vi "Testing.vi"() -> ()   [LabVIEW 2016, in "User Interface.lvlib"]
uses:
  User Interface.lvlib
  <vilib>/Utility/miscctls.llb/LVPointTypeDef.ctl
  Testing Command.ctl
  VI Name.ctl
panel:
  in  "EXIT":bool
  out "error out":errorcluster
  in  "error in (no error)":errorcluster
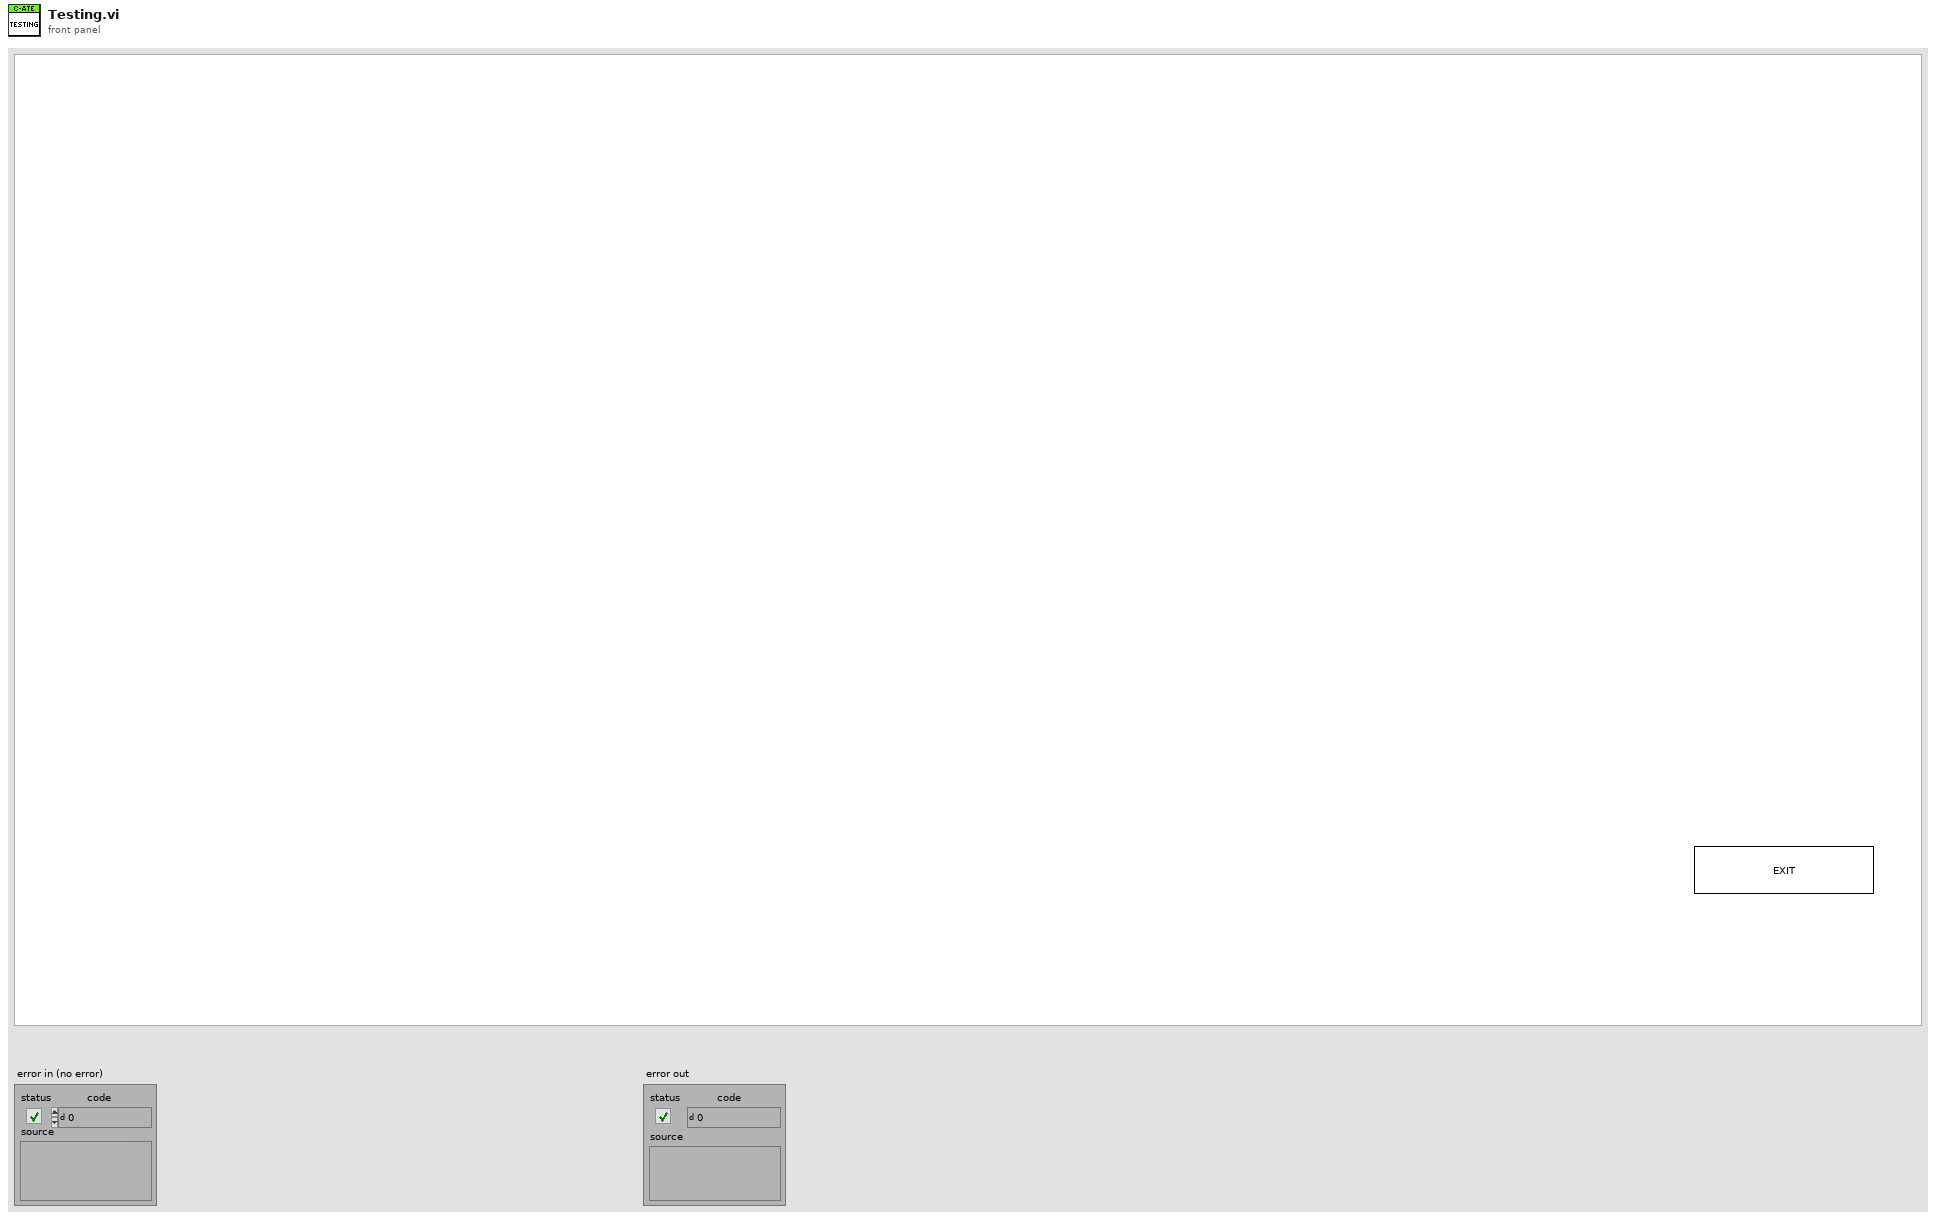
[diagram p1: front panel]
types:
  T1 = typedef "User Interface.lvlib/Testing Command.ctl" = enum16{"Init", "Main", "Close"}
  T2 = typedef "LVPointTypeDef.ctl" = cluster{"Horizontal":i16, "Vertical":i16}
  T3 = typedef "User Interface.lvlib/VI Name.ctl" = enum16{"Dashboard", "Maintenance", "Recipe", "Inst Configuration", "Testing", "Report"}
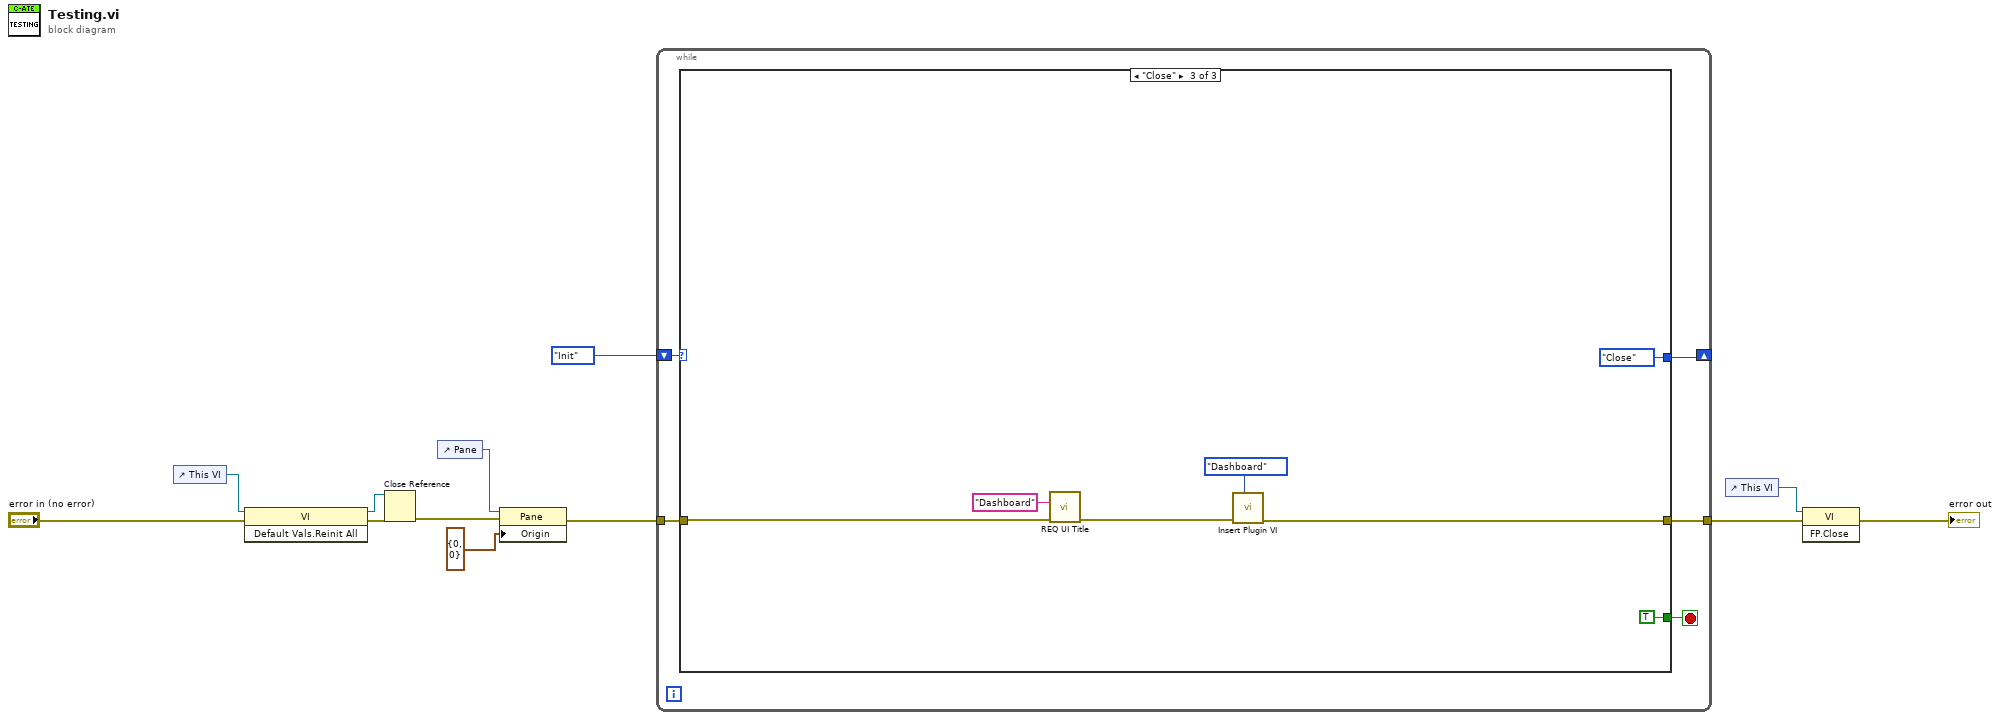
[diagram p0: block diagram]
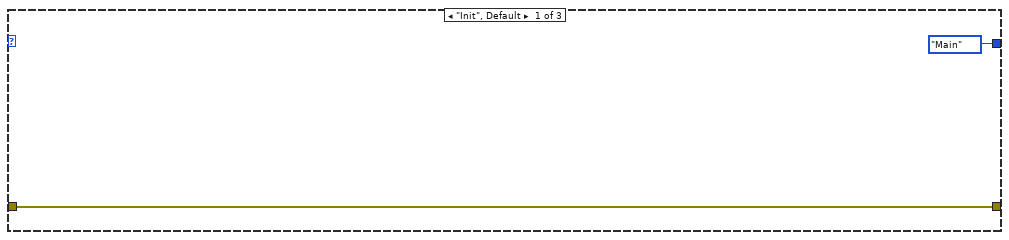
[diagram p2: hidden frame]
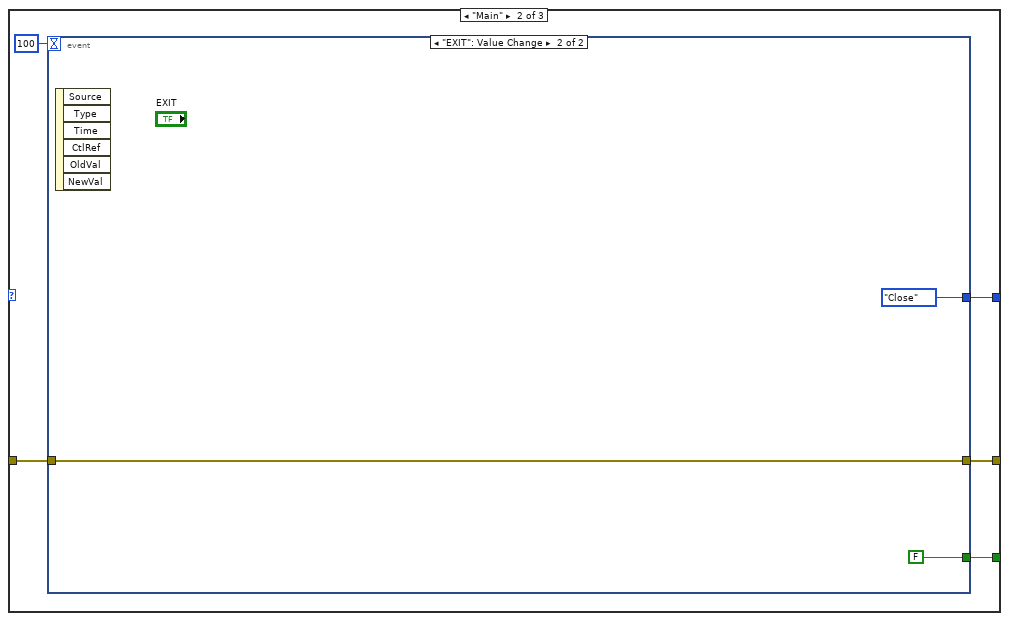
[diagram p3: hidden frame]
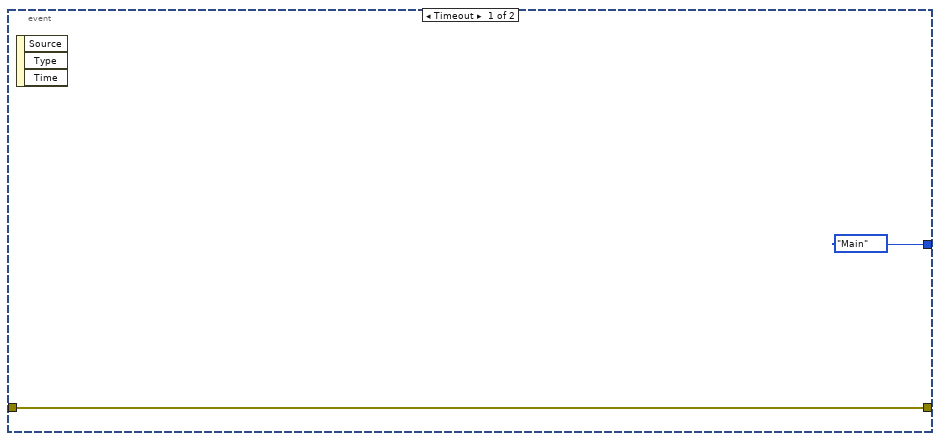
[diagram p4: hidden frame]
diagram:
  n1 = control-ref of="This VI"() -> (w7:refnum<vi>)
  n2 = invoke class="VI" method="Default Vals.Reinit All"(reference=w7, error in="error in (no error)") -> (reference out=w5:refnum<vi>, error out=w6:errorcluster)  [unwired: 1 in, 1 out]
  n3 = Close Reference(reference=w5, error in (no error)=w6) -> (error out=w3:errorcluster)
  n4 = control-ref of="Pane"() -> (w2:refnum<vi>)
  n5 = property class="Pane"(reference=w2, error in=w3, "Origin"=T2 {"Horizontal"=0, "Vertical"=0}) -> (error out=w12:errorcluster)  [unwired: 1 out]
  n6 = while {
    tunnel: w12 -> [w17]
    shift-right: [w13] -> _
    shift-left: Testing_Command."Init" -> [w16]
    tunnel: [w15] -> w9
    stop <- w14 stop-if-true
    n7 = case shown="\"Close\"" w16 {
      tunnel: w17 -> [w19 w23 w31]
      tunnel: [w19 w22 w35] -> w15
      tunnel: [_ w21 TRUE] -> w14
      tunnel: [Testing_Command."Main" w20 Testing_Command."Close"] -> w13
      frame "Init", Default {
      }
      frame "Main" {
        n8 = event shown="[1] \"EXIT\": Value Change" {
          selector: _ -> [_ _]
          dyn-events: _ -> [_ _]
          timeout: 100 -> [_ _]
          tunnel: w23 -> [w26 w29]
          tunnel: [w26 w29] -> w22
          tunnel: [_ FALSE] -> w21
          tunnel: [Testing_Command."Main" ("Command") Testing_Command."Close"] -> w20
          event Timeout {
            n9 = event-data() -> ()  [unwired: 1 in, 3 out]
          }
          event "EXIT": Value Change {
            n10 = event-data() -> ()  [unwired: 1 in, 6 out]
          }
        }
      }
      frame "Close" {
        n11 = call "REQ UI Title.vi"("error in"=w31, "UI Title"="Dashboard" ("ATE Title")) -> ("error out"=w30:errorcluster)  [unwired: 9 in]
        n12 = call "Insert Plugin VI.vi"("VI Name"=VI_Name."Dashboard", "error in (no error)"=w30) -> ("error out"=w35:errorcluster)  [unwired: 9 in]
      }
    }
  }
  n13 = control-ref of="This VI"() -> (w10:refnum<vi>)
  n14 = invoke class="VI" method="FP.Close"(reference=w10, error in=w9) -> (error out=→"error out":errorcluster)  [unwired: 1 in, 2 out]
